vi "RedGreenBlueExample.vi"() -> ()   [LabVIEW 2012]
uses:
  Local Settings/Temporary Internet Files/Content.IE5/80YCGHAB/forum nov 12 red green blue.ctl
panel:
  in  "stop":bool
  out "Current State":T1
  in  "Numeric":i32
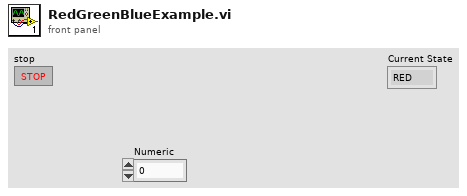
[diagram p1: front panel]
types:
  T1 = typedef "Control 3" = enum16{"RED", "GREEN", "BLUE"}
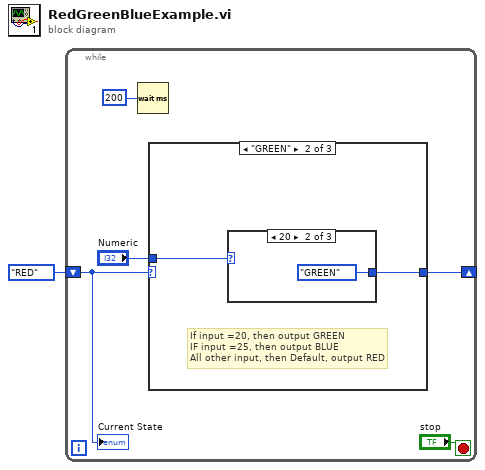
[diagram p0: block diagram]
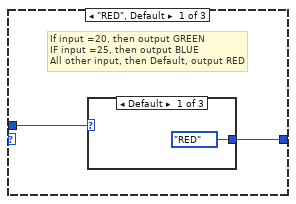
[diagram p2: hidden frame]
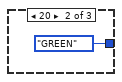
[diagram p3: hidden frame]
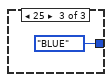
[diagram p4: hidden frame]
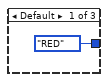
[diagram p5: hidden frame]
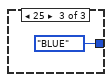
[diagram p6: hidden frame]
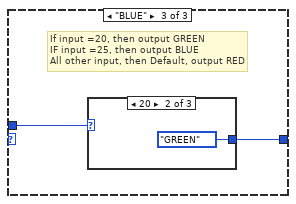
[diagram p7: hidden frame]
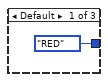
[diagram p8: hidden frame]
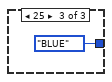
[diagram p9: hidden frame]
diagram:
  n1 = while {
    shift-right: [w4] -> _
    shift-left: Control_3."RED" -> [w6]
    stop <- "stop" stop-if-true
    n2 = Wait (ms)(milliseconds to wait=u32 200) -> ()  [unwired: 1 out]
    n3 = case shown="\"GREEN\"" w6 {
      tunnel: "Numeric" -> [w7 w13 w17]
      tunnel: [w8 w12 w18] -> w4
      frame "RED", Default {
        # "If input =20, then output GREEN\nIF input =25, then output BLUE\nAll other input, then Default, output RED"
        n4 = case shown="Default" w7 {
          tunnel: [Control_3."RED" Control_3."GREEN" Control_3."BLUE"] -> w8
          frame Default {
          }
          frame 20 {
          }
          frame 25 {
          }
        }
      }
      frame "GREEN" {
        # "If input =20, then output GREEN\nIF input =25, then output BLUE\nAll other input, then Default, output RED"
        n5 = case shown="20" w13 {
          tunnel: [Control_3."RED" Control_3."GREEN" Control_3."BLUE"] -> w12
          frame Default {
          }
          frame 20 {
          }
          frame 25 {
          }
        }
      }
      frame "BLUE" {
        # "If input =20, then output GREEN\nIF input =25, then output BLUE\nAll other input, then Default, output RED"
        n6 = case shown="20" w17 {
          tunnel: [Control_3."RED" Control_3."GREEN" Control_3."BLUE"] -> w18
          frame Default {
          }
          frame 20 {
          }
          frame 25 {
          }
        }
      }
    }
    "Current State" <- w6
  }
